vi "Add_new_Columns_to_file.vi"(0 "Filename":path, 5 "Extra Chs":string[](array[string]), 9 "New Ch data":string[][](array[string]), 11 "Start of read offset (chars.: 0)":i32) -> ()   [LabVIEW 2010]
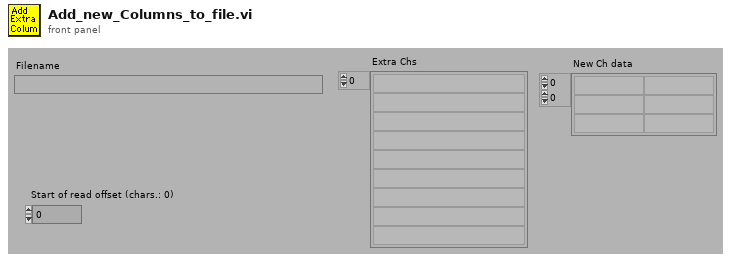
[diagram p1: front panel]
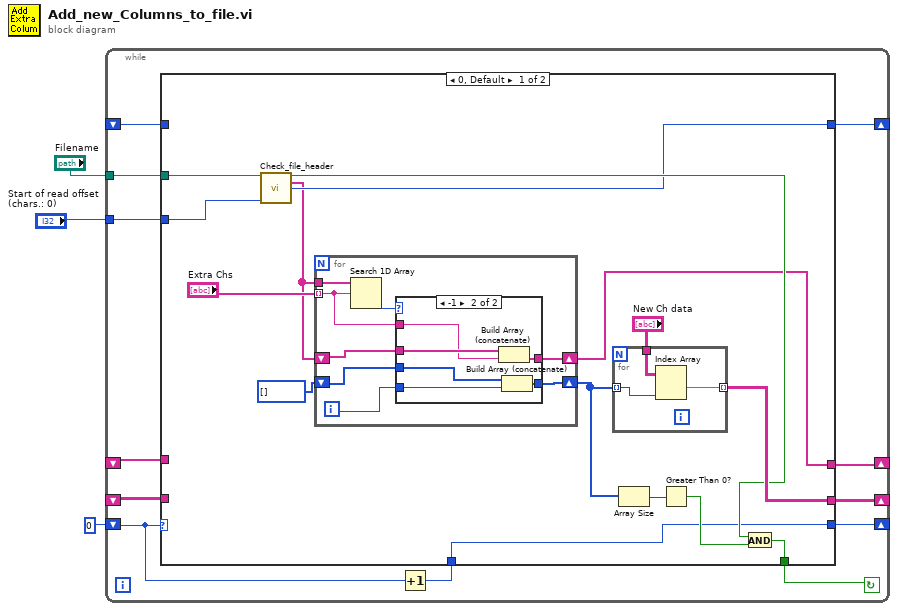
[diagram p0: block diagram]
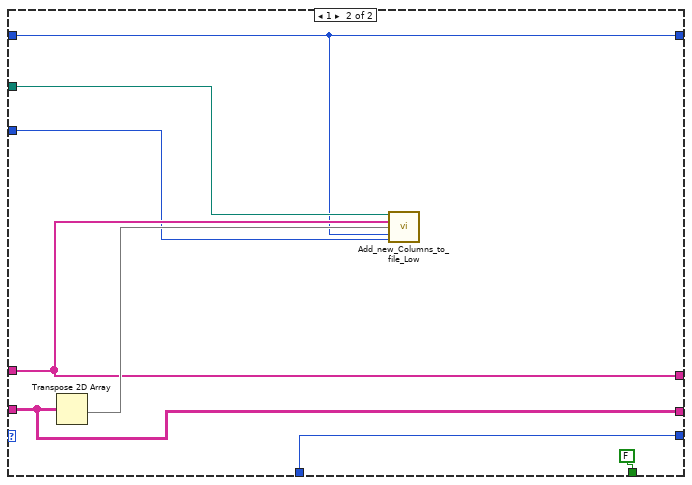
[diagram p3: hidden frame]
diagram:
  n1 = while {
    shift-left: _ -> [w4]
    shift-right: [w5] -> _
    tunnel: "Start of read offset (chars.: 0)" -> [w6]
    tunnel: "Filename" -> [w12]
    shift-left: _ -> [w11]
    shift-right: [w13] -> _
    shift-left: _ -> [w10]
    shift-right: [w14] -> _
    shift-left: 0 -> [w9]
    shift-right: [w7] -> _
    stop <- w15 continue-if-true
    n2 = Increment(x=w9) -> (x+1=w8:i32)
    n3 = case shown="0, Default" w9 {
      tunnel: [w16 FALSE] -> w15
      tunnel: [w27 w53] -> w14
      tunnel: [w17 w52] -> w13
      tunnel: w12 -> [w22 w57]
      tunnel: w11 -> [_ w52]
      tunnel: w10 -> [_ w53]
      tunnel: w8 -> [w21 w54]
      tunnel: [w21 w54] -> w7
      tunnel: w6 -> [w20 w51]
      tunnel: [w19 w50] -> w5
      tunnel: w4 -> [_ w50]
      frame 0, Default {
        n4 = call "Check_file_header.vi"("Filename"=w22, "Start of read offset (chars.: 0)"=w20) -> ("exists?"=w23:bool, "Merged Channels"=w18:string[], "Start of data (bytes)"=w19:i32)  [unwired: 7 in, 4 out]
        n5 = for {
          tunnel: "Extra Chs" -> [w34] mode=indexing
          tunnel: w18 -> [w41]
          shift-right: [w38] -> w17
          shift-left: w18 -> [w39]
          shift-right: [w35] -> w26
          shift-left: i32[] [] -> [w37]
          i -> [w36]
          n6 = Search 1D Array(1D array=w41, element=w34) -> (index of element=w40:i32)  [unwired: 1 in]
          n7 = case shown="-1" w40 {
            tunnel: w39 -> [w43 w49]
            tunnel: [w43 w48] -> w38
            tunnel: w34 -> [_ w47]
            tunnel: w37 -> [w42 w46]
            tunnel: w36 -> [_ w45]
            tunnel: [w42 w44] -> w35
            frame 0, Default {
            }
            frame -1 {
              n8 = Build Array (concatenate)(w49, w47) -> (w48:string[])
              n9 = Build Array (concatenate)(w46, w45) -> (w44:i32[])
            }
          }
        }
        n10 = for {
          tunnel: w26 -> [w31] mode=indexing
          tunnel: "New Ch data" -> [w33]
          tunnel: [w32] -> w27 mode=indexing
          n11 = Index Array(array=w33, index (col)=w31) -> (element=w32:string[])  [unwired: 1 in]
        }
        n12 = Array Size(array=w26) -> (size(s)=w25:i32)
        n13 = Greater Than 0?(x=w25) -> (x > 0?=w24:bool)
        n14 = And(x=w23, y=w24) -> (x .and. y?=w16:bool)
      }
      frame 1 {
        n15 = Transpose 2D Array(2D array=w53) -> (transposed array=w56:string[][])
        n16 = call "Add_new_Columns_to_file_Low.vi"("Filename"=w57, "Merged Channels"=w52, "String to add"=w56, "Start of data (bytes)"=w50, "Start of read offset (chars.: 0)"=w51) -> ()  [unwired: 11 in]
      }
    }
  }
